vi "deadband.vi"(4 "Deadband":dbl, 5 "D":dbl, 6 "C":dbl, 7 "B":dbl, 8 "A":dbl) -> (0 "mD":dbl, 1 "mC":dbl, 2 "mB":dbl, 3 "mA":dbl)   [LabVIEW 2010, in "LASA Beta.lvrbt"]
doc: "Takes normalized input`s absolute value and sets it to 0 if less than or equal to deadband constant.\n\n<b>Inputs </b>\n<b>A-D </b> are normalized inputs.\n<b>Deadband </b> is the deadband constant.\n\n<b>Outputs </b>\n<b>mA-mD </b> are either equal to <b>A-D </b> or 0 if their absolute values were originally less than or equal to the deadband value"
uses:
  LASA Beta.lvrbt
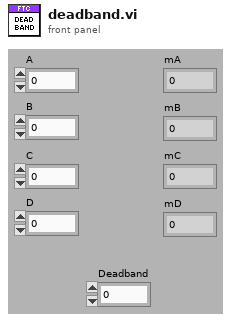
[diagram p1: front panel]
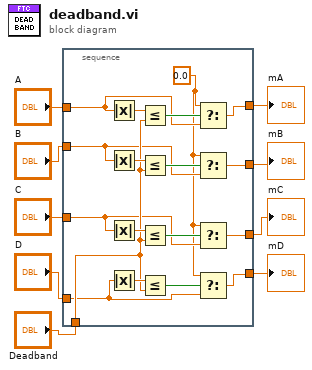
[diagram p0: block diagram]
diagram:
  n1 = stacked-sequence {
    tunnel: "Deadband" -> [w19]
    tunnel: "D" -> [w18]
    tunnel: "C" -> [w17]
    tunnel: "B" -> [w16]
    tunnel: "A" -> [w15]
    tunnel: [w13] -> w4
    tunnel: [w12] -> w3
    tunnel: [w11] -> w2
    tunnel: [w10] -> w1
    frame #0 {
      w14 = 0.0 ("t")
      n2 = Absolute Value(x=w15) -> (abs(x)=w22:dbl)
      n3 = Absolute Value(x=w16) -> (abs(x)=w23:dbl)
      n4 = Absolute Value(x=w17) -> (abs(x)=w21:dbl)
      n5 = Absolute Value(x=w18) -> (abs(x)=w20:dbl)
      n6 = Less Or Equal?(x=w22, y=w19) -> (x <= y?=w27:bool)
      n7 = Less Or Equal?(x=w23, y=w19) -> (x <= y?=w26:bool)
      n8 = Less Or Equal?(x=w21, y=w19) -> (x <= y?=w25:bool)
      n9 = Less Or Equal?(x=w20, y=w19) -> (x <= y?=w24:bool)
      n10 = Select(t=w14, s=w27, f=w15) -> (s? t:f=w13:dbl)
      n11 = Select(t=w14, s=w26, f=w16) -> (s? t:f=w12:dbl)
      n12 = Select(t=w14, s=w25, f=w17) -> (s? t:f=w11:dbl)
      n13 = Select(t=w14, s=w24, f=w18) -> (s? t:f=w10:dbl)
    }
  }
  "mA" <- w4
  "mB" <- w3
  "mC" <- w2
  "mD" <- w1
